vi "Simulator PWM Calibrate.vi"(8 "error in (no error)":errorcluster, 10 "Normalize? (T)":T1) -> (0 "error out":errorcluster {"code" format="%.0x"}, 3 "Normalized?":T1)   [LabVIEW 2011]
uses:
  PWM Normalization State.ctl
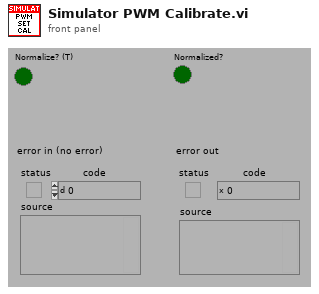
[diagram p1: front panel]
types:
  T1 = typedef "PWM Normalization State.ctl" = bool
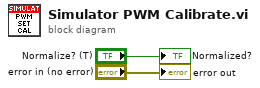
[diagram p0: block diagram]
diagram:
  "error out" <- "error in (no error)"
  "Normalized?" <- "Normalize? (T)"
